vi "Test HovaCAL Start Kondition.vi"(8 "Fehler (Eingang, kein Fehler)":errorcluster, 11 "Sprachliste":string[][](array[string])) -> (0 "Fehler (Ausgang)":errorcluster, 3 "ok":bool)   [LabVIEW 2020, in "EPA 1065.lvlib" / "HovaCAL Interference verificaton.lvlib"]
uses:
  HovaCAL Interference verificaton.lvlib
  Aktion FGV Interference.ctl
  Linearisierung V2/Gasteiler/HovaCAL_Interface/Kommunikation/Aktion_FGV_HovaCAL_Interface_GetData.ctl
  Linearisierung V2/Gasteiler/HovaCAL_Interface/Kommunikation/Kommunikation.lvlib
  Sprachverwaltung/Sprachverwaltung.lvlib
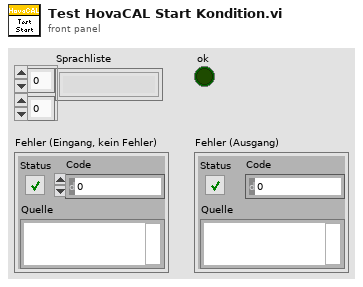
[diagram p1: front panel]
types:
  T1 = typedef "Linearisierung v2.lvlib/Gasteiler.lvlib/HovaCAL_Interface.lvlib/Kommunikation.lvlib/Aktion_FGV_HovaCAL_Interface_GetData.ctl" = enum16{"lesen", "SystemInfo", "MFC Info", "actual Values", "Limits", "first contact"}
  T2 = typedef "EPA 1065.lvlib/HovaCAL Interference verificaton.lvlib/Aktion FGV Interference.ctl" = enum16{"Lesen", "TestKonfig", "TestSetting", "Einheiten", "Ergebnis", "Laden", "Tabelle", "Speichern", "löschen"}
  T3 = typedef "EPA 1065.lvlib/HovaCAL Interference verificaton.lvlib/TestKonfig.ctl" = cluster{"TestKonfig H2O":T4, "TestKonfig Interferent":T10}
  T4 = typedef "EPA 1065.lvlib/HovaCAL Interference verificaton.lvlib/TestKonfig H2O.ctl" = cluster{"Modus":T5, "Komponente:":u16, "Eingangs Konzentration:":dbl, "Einheit":T6, "Anzahl Stufen":sgl, "Zeitdauer Stufen":sgl, "Max Fehler":sgl, "zusätzliche Zeitdauer Erster Punkt":sgl, "Punkte umkehren":bool, "Stufen Tabelle":T7, "HovaCAL Flow Input Cluster":T8, "HovaCAL Temperature":T9}
  T5 = typedef "EPA 1065.lvlib/HovaCAL Interference verificaton.lvlib/Modus.ctl" = u16
  T6 = typedef "Linearisierung v2.lvlib/SpanEinstellungen.lvlib/Einheit.ctl" = enum16{"ppm", "%"}
  T7 = typedef "Linearisierung v2.lvlib/Gasteiler.lvlib/Stufen Tabelle.ctl" = string[][]
  T8 = typedef "Linearisierung v2.lvlib/Gasteiler.lvlib/HovaCAL_Interface.lvlib/Controls.lvlib/Flow Einstellung.ctl" = cluster{"HovaCAL Flow Input Cluster":dbl}
  T9 = typedef "Linearisierung v2.lvlib/Gasteiler.lvlib/HovaCAL_Interface.lvlib/Controls.lvlib/Temp Sollwerte Anzeige.ctl" = dbl[]
  T10 = typedef "EPA 1065.lvlib/HovaCAL Interference verificaton.lvlib/TestKonfig Interferents.ctl" = cluster{"MFC1":enum16{"MFC 1"}, "Eingangs Konzentration MFC1":dbl, "Einheit MFC1 Eingang":T6, "Ausgangs Konzentration MFC1":dbl, "Einheit MFC1 Ausgang":T6, "MFC2":T11, "Referenz-Interferent:":u16, "Gasflaschen Nr MFC2":string, "Accuracy MFC2":string, "Eingangs Konzentration MFC2":dbl, "Einheit MFC2 Eingang":T6, "Ausgangs Konzentration MFC2":dbl, "Einheit MFC2 Ausgang":T6, "MFC3":T11, "Kontroll-Interferent:":u16, "Gasflaschen Nr MFC3":string, "Accuracy MFC3":string, "Eingangs Konzentration MFC3":dbl, "Einheit MFC3 Eingang":T6, "Ausgangs Konzentration MFC3":dbl, "Einheit MFC3 Ausgang":T6, "Gasflasche MFC2":T12, "Gasflasche MFC3":T12}
  T11 = typedef "EPA 1065.lvlib/HovaCAL Interference verificaton.lvlib/MFCAuswahl.ctl" = u16
  T12 = typedef "System Einstellungen V2.lvlib/Gasflasche Auswahl.ctl" = u16
  T13 = typedef "Linearisierung v2.lvlib/Gasteiler.lvlib/HovaCAL_Interface.lvlib/Controls.lvlib/Info Cluster.ctl" = cluster{"device":string, "version":string, "number of mfc":i32, "number of pumps":i32, "number of temp controllers":i32, "number of mfs":i32, "number of balances":i32}
  T14 = cluster{"temp SP":dbl, "temp":dbl, "humidity":dbl}[]
  T15 = cluster{"temp SP":dbl, "temp":dbl, "humidity":dbl}
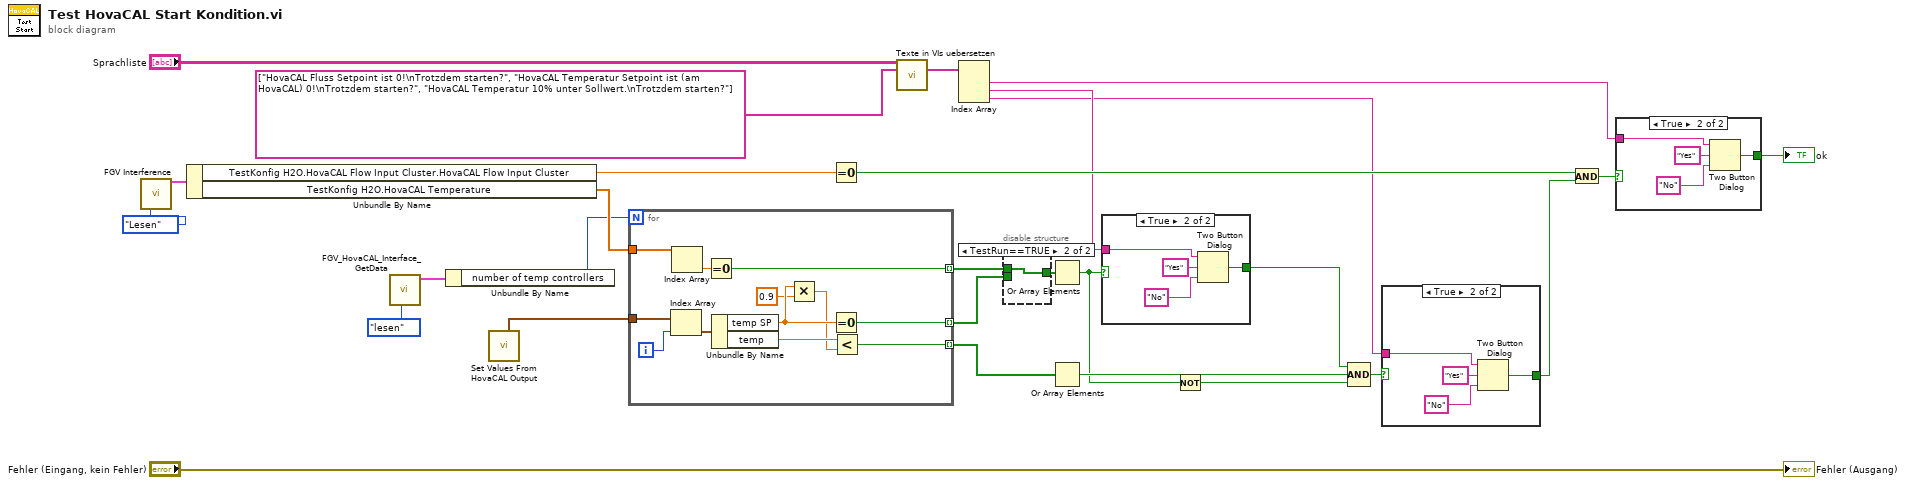
[diagram p0: block diagram]
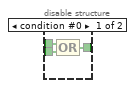
[diagram p2: hidden frame]
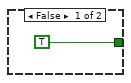
[diagram p3: hidden frame]
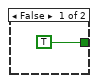
[diagram p4: hidden frame]
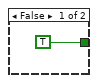
[diagram p5: hidden frame]
diagram:
  n1 = call "FGV Interference.vi"("Aktion FGV Interference"=Aktion_FGV_Interference."Lesen") -> ("TestKonfig"=w21:T3)  [unwired: 9 in, 5 out]
  n2 = Unbundle By Name(w21) -> ("TestKonfig H2O.HovaCAL Flow Input Cluster.HovaCAL Flow Input Cluster"=w27:dbl, "TestKonfig H2O.HovaCAL Temperature"=w28:T9)
  n3 = call "FGV_HovaCAL_Interface_GetData.vi"("Aktion"=Aktion_FGV_HovaCAL_Interface_GetData."lesen") -> ("System Cluster out"=w24:T13)  [unwired: 6 in, 4 out]
  n4 = Unbundle By Name(w24) -> ("number of temp controllers"=w25:i32)
  n5 = call "Set Values From HovaCAL Output.vi"() -> ("Cluster.Temp Cluster"=w26:T14)  [unwired: 2 in, 9 out]
  n6 = for {
    N: w25 -> [_]
    tunnel: w26 -> [w40]
    tunnel: w28 -> [w37]
    tunnel: [w35] -> w20 mode=indexing
    tunnel: [w30] -> w19 mode=indexing
    tunnel: [w29] -> w10 mode=indexing
    i -> [w39]
    n7 = Index Array(array=w40, index=w39) -> (element=w38:T15)
    n8 = Index Array(array=w37) -> (element=w36:dbl)  [unwired: 1 in]
    n9 = Equal To 0?(x=w36) -> (x = 0?=w35:bool)
    n10 = Unbundle By Name(w38) -> ("temp SP"=w33:dbl, "temp"=w34:dbl)
    n11 = Multiply(x=w33, y=0.9) -> (x*y=w31:dbl)
    n12 = Equal To 0?(x=w33) -> (x = 0?=w30:bool)
    n13 = Less?(x=w34, y=w31) -> (x < y?=w29:bool)
  }
  n14 = Equal To 0?(x=w27) -> (x = 0?=w14:bool)
  n15 = call "Texte in VIs uebersetzen.vi"("Sprachliste"="Sprachliste", "String-Array zum Übersetzen"=string[] ["HovaCAL Fluss Setpoint ist 0!\nTrotzdem starten?", "HovaCAL Temperatur Setpoint ist (am HovaCAL) 0!\nTrotzdem starten?", "HovaCAL Temperatur 10% unter Sollwert.\nTrotzdem starten?"] ("Nachricht")) -> ("String-Array zum Übersetzen"=w16:string[])  [unwired: 9 in, 4 out]
  n16 = Index Array(array=w16) -> (element #1=w13:string, element #2=w12:string, element #3=w9:string)  [unwired: 3 in]
  n17 = disable-structure shown="TestRun==TRUE" {
    disable-tunnel: w20 -> [w43 w44]
    disable-tunnel: w19 -> [w42 _]
    disable-tunnel: [w41 w44] -> w15
    frame condition #0 {
      n18 = Compound Arithmetic op=OR ("Mehrfacharithmetik")(w43, w42) -> (w41:bool[])
    }
    frame condition #1 (active) {
    }
  }
  n19 = Or Array Elements(Boolean array=w15) -> (logical OR=w7:bool)
  n20 = Or Array Elements(Boolean array=w10) -> (logical OR=w11:bool)
  n21 = case shown="True" w7 {
    tunnel: w12 -> [_ w47]
    tunnel: [TRUE ("T button?") w46] -> w5
    frame False {
    }
    frame True {
      n22 = Two Button Dialog(message=w47, 1:"No" ("Text für F-Schaltfläche (\"Abbrechen\")"), 2:"Yes" ("Text für T-Schaltfläche (\"OK\")")) -> (T button?=w46:bool)
    }
  }
  n23 = Not(x=w7) -> (.not. x?=w6:bool)
  n24 = Compound Arithmetic op=AND ("Mehrfacharithmetik")(w5, w11, w6) -> (w8:bool)
  n25 = case shown="True" w8 {
    tunnel: w9 -> [_ w52]
    tunnel: [TRUE ("T button?") w51] -> w3
    frame False {
    }
    frame True {
      n26 = Two Button Dialog(message=w52, 1:"No" ("Text für F-Schaltfläche (\"Abbrechen\")"), 2:"Yes" ("Text für T-Schaltfläche (\"OK\")")) -> (T button?=w51:bool)
    }
  }
  n27 = And(x=w14, y=w3) -> (x .and. y?=w4:bool)
  n28 = case shown="True" w4 {
    tunnel: w13 -> [_ w57]
    tunnel: [TRUE ("T button?") w56] -> w2
    frame False {
    }
    frame True {
      n29 = Two Button Dialog(message=w57, 1:"No" ("Text für F-Schaltfläche (\"Abbrechen\")"), 2:"Yes" ("Text für T-Schaltfläche (\"OK\")")) -> (T button?=w56:bool)
    }
  }
  "ok" <- w2
  "Fehler (Ausgang)" <- "Fehler (Eingang, kein Fehler)"
